vi "DataCleanUp.vi"(9 "Data in":string[](array[string]), 10 "Team":string) -> (1 "Data out":string[](array[string]))   [LabVIEW 2017]
uses:
  <vilib>/Utility/config.llb/Write Key (String).vi
  <vilib>/regexp/Match Regular Expression.xnode
  <vilib>/Utility/config.llb/NI_LVConfig.lvlib
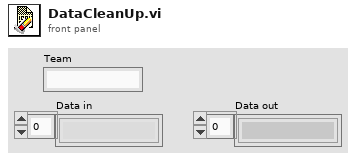
[diagram p1: front panel]
types:
  T1 = typedef "NI_LVConfig.lvlib/Config Data RefNum.ctl" = refnum<k1>
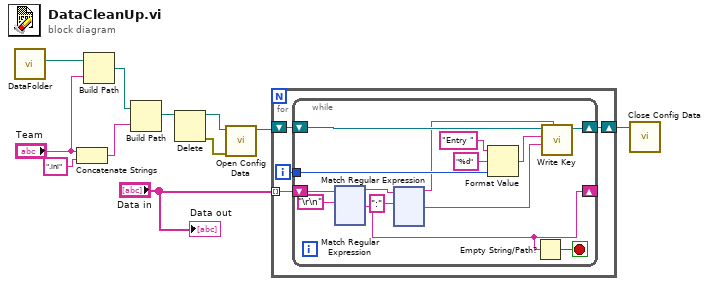
[diagram p0: block diagram]
diagram:
  n1 = call "DataFolder.vi"() -> ("appended path"=w11:path)  [unwired: 11 in]
  n2 = Concatenate Strings("Team", ".ini" ("format string")) -> (w9:string)
  n3 = Build Path(base path=w11, name or relative path="Team") -> (appended path=w8:path)
  n4 = Build Path(base path=w8, name or relative path=w9) -> (appended path=w7:path)
  n5 = Delete(path (use dialog)=w7) -> (deleted path=w5:path, error out=w6:errorcluster)  [unwired: 4 in, 1 out]
  n6 = call <vilib>:"Open Config Data.vi"("error in (no error)"=w6, "configuration file path"=w5) -> ("refnum"=w4:T1)  [unwired: 7 in, 2 out]
  n7 = for {
    tunnel: "Data in" -> [w12] mode=indexing
    shift-right: [w13] -> w2
    shift-left: w4 -> [w15]
    i -> [w14]
    n8 = while {
      tunnel: w14 -> [w28]
      shift-right: [w27] -> w13
      shift-left: w15 -> [w29]
      shift-right: [w16] -> _
      shift-left: w12 -> [w26]
      stop <- w17 stop-if-true
      n9 = xnode "Match Regular Expression"("input string"=w26, "regular expression"="\r\n") -> ("before match"=w25:string, "after match"=w16:string)  [unwired: 4 in, 3 out]
      n10 = xnode "Match Regular Expression"("input string"=w25, "regular expression"=":") -> ("before match"=w22:string, "after match"=w21:string)  [unwired: 4 in, 3 out]
      n11 = Format Value(string ("")="Entry ", format string="%d", value (0)=w28) -> (output string=w18:string)
      n12 = Empty String/Path?(string/path=w16) -> (empty?=w17:bool)
      n13 = call-poly <vilib>:"Write Key.vi"("section"=w22, "value"=w21, "key"=w18, "refnum"=w29) -> ("refnum out"=w27:T1)  [unwired: 5 in, 2 out]
    }
  }
  n14 = call <vilib>:"Close Config Data.vi"("refnum"=w2) -> ()  [unwired: 9 in, 2 out]
  "Data out" <- "Data in"
